vi "Compute Gyro Turn.vi"(8 "error in (no error)":errorcluster, 10 "Negate stuff":bool, 11 "Turn? Right Positive.":dbl) -> (0 "error out":errorcluster, 2 "Right Drive":dbl, 3 "Left drive":dbl, 5 "done":bool)   [LabVIEW 2017]
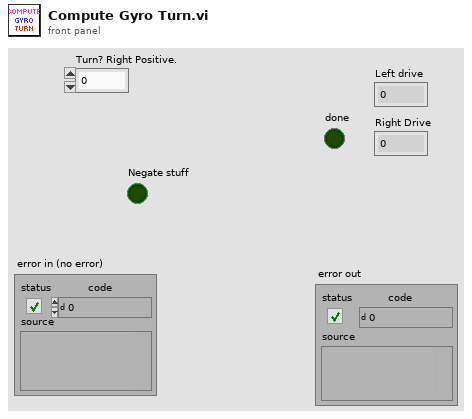
[diagram p1: front panel]
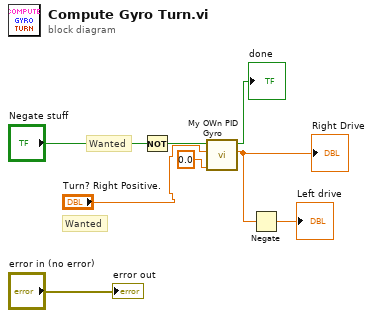
[diagram p0: block diagram]
diagram:
  # "Wanted"
  # "Wanted"
  n1 = Not(x="Negate stuff") -> (.not. x?=w3:bool)
  n2 = call "My OWn PID Gyro.vi"("Current Input"=0.0, "Wanted End"="Turn? Right Positive.", "Negate Stuff"=w3) -> ("Output"=w5:dbl, "Done"=→"done":bool)  [unwired: 7 in]
  "Right Drive" <- w5
  n3 = Negate(x=w5) -> (-x=→"Left drive":dbl)
  "error out" <- "error in (no error)"
